vi "Sweep_Test.vi"() -> ()   [LabVIEW 2026]
panel:
  out "Gain vs Frequency":cluster{dbl[], dbl[]}(graph)
  in  "Step (MHz)":dbl
  in  "Stop (MHz)":dbl
  in  "Start (MHz)":dbl
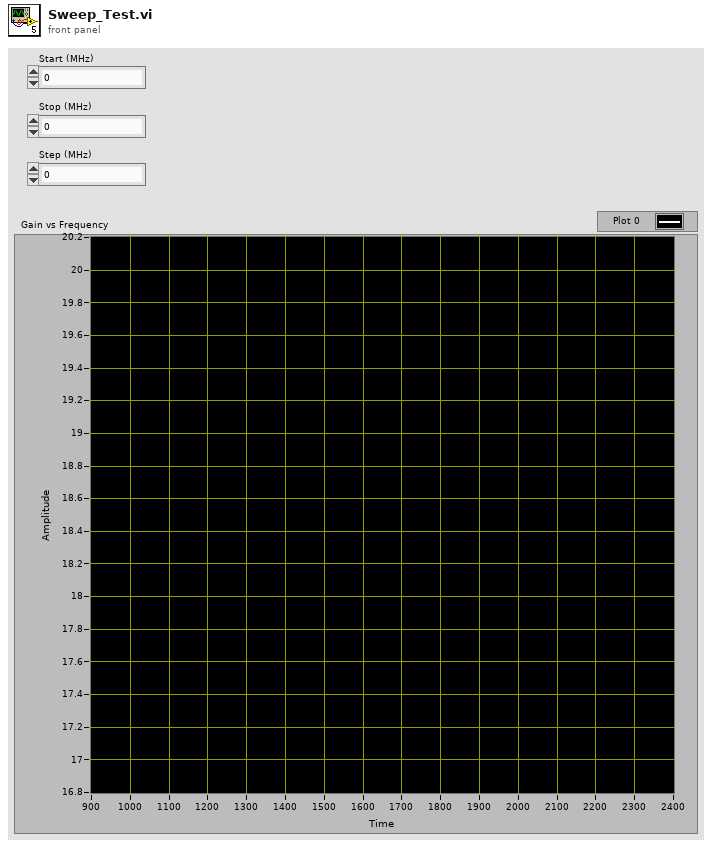
[diagram p1: front panel]
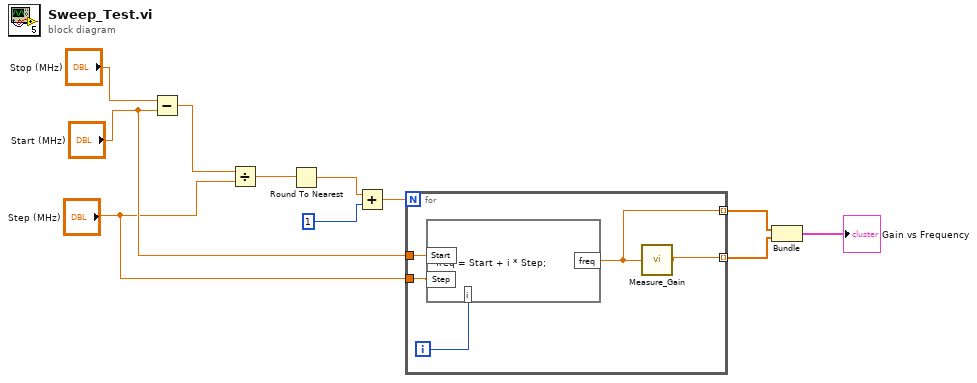
[diagram p0: block diagram]
diagram:
  n1 = Subtract(x="Stop (MHz)", y="Start (MHz)") -> (x-y=w10:dbl)
  n2 = Divide(x=w10, y="Step (MHz)") -> (x/y=w9:dbl)
  n3 = Round To Nearest(number=w9) -> (nearest integer value=w8:dbl)
  n4 = Add(x=w8, y=1) -> (x+y=w6:dbl)
  n5 = for {
    N: w6 -> [_]
    tunnel: "Start (MHz)" -> [w16]
    tunnel: "Step (MHz)" -> [w15]
    tunnel: [w13] -> w2 mode=indexing
    tunnel: [w12] -> w3 mode=indexing
    i -> [w14]
    n6 = formula code="freq = Start + i * Step;"("Start"=w16, "Step"=w15, "i"=w14) -> ("freq"=w12:dbl)
    n7 = call "Measure_Gain.vi"("Frequency (MHz)"=w12) -> ("Gain (dB)"=w13:dbl)
  }
  n8 = Bundle(w3, w2) -> (→"Gain vs Frequency":cluster{dbl[], dbl[]})  [unwired: 1 in]
